vi "VI Tree.vi"   [LabVIEW 2016]
uses:
  Attributes.vi
  Error Code File Properties.ctl
  Error Owner and ID.ctl
  Error Owners and IDs.ctl
  Scope.ctl
types:
  T1 = typedef "Scope.ctl" = enum16{"project", "global"}
  T2 = typedef "Error Owners and IDs.ctl" = cluster{"owner path":string, "error IDs":string[]}
  T3 = typedef "Error Owner and ID.ctl" = cluster{"owner path":string, "ID":string}
  T4 = typedef "Error Code File Properties.ctl" = cluster{"path":path, "simplified path":string, "name":string, "display name":string, "family name":string, "comment":string, "parsable?":bool, "file modified?":bool}
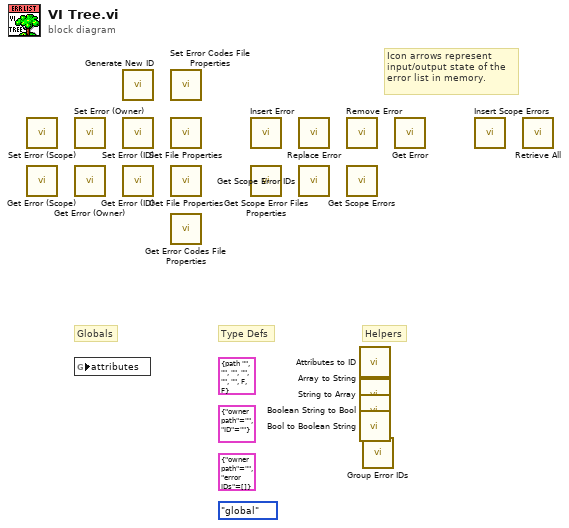
[diagram p0: block diagram]
diagram:
  (unwired) Scope."global" ("scope")
  (unwired) T2 {"owner path"="", "error IDs"=[]} ("error owners and IDs")
  (unwired) T3 {"owner path"="", "ID"=""} ("error owner and ID")
  (unwired) T4 {"path"=path "", "simplified path"="", "name"="", "display name"="", "family name"="", "comment"="", "parsable?"=FALSE, "file modified?"=FALSE} ("error code file properties")
  # "Icon arrows represent input/output state of the error list in memory."
  # "Globals"
  # "Type Defs"
  # "Helpers"
  n1 = call "Set Error (Scope).vi"() -> ()  [unwired: 10 in, 2 out]
  n2 = call "Get Error (Scope).vi"() -> ()  [unwired: 8 in, 4 out]
  n3 = call "Set Error (Owner).vi"() -> ()  [unwired: 10 in, 2 out]
  n4 = call "Get Error (Owner).vi"() -> ()  [unwired: 8 in, 4 out]
  n5 = global read "Attributes.vi" "attributes"() -> ()  [unwired: 1 in]
  n6 = call "Generate New ID.vi"() -> ()  [unwired: 9 in, 3 out]
  n7 = call "Set Error (ID).vi"() -> ()  [unwired: 10 in, 2 out]
  n8 = call "Get Error (ID).vi"() -> ()  [unwired: 7 in, 5 out]
  n9 = call "Set Error Codes File Properties.vi"() -> ()  [unwired: 10 in, 2 out]
  n10 = call "Set File Properties.vi"() -> ()  [unwired: 10 in, 2 out]
  n11 = call "Get File Properties.vi"() -> ()  [unwired: 9 in, 3 out]
  n12 = call "Get Error Codes File Properties.vi"() -> ()  [unwired: 8 in, 4 out]
  n13 = call "Insert Error.vi"() -> ()  [unwired: 10 in, 2 out]
  n14 = call "Get Scope Error Files Properties.vi"() -> ()  [unwired: 7 in, 5 out]
  n15 = call "Replace Error.vi"() -> ()  [unwired: 10 in, 2 out]
  n16 = call "Get Scope Error IDs.vi"() -> ()  [unwired: 9 in, 3 out]
  n17 = call "Remove Error.vi"() -> ()  [unwired: 10 in, 2 out]
  n18 = call "Get Scope Errors.vi"() -> ()  [unwired: 7 in, 5 out]
  n19 = call "Attributes to ID.vi"() -> ()  [unwired: 1 in, 1 out]
  n20 = call "Array to String.vi"() -> ()  [unwired: 2 in, 1 out]
  n21 = call "String to Array.vi"() -> ()  [unwired: 2 in, 1 out]
  n22 = call "Boolean String to Bool.vi"() -> ()  [unwired: 1 in, 1 out]
  n23 = call "Bool to Boolean String.vi"() -> ()  [unwired: 1 in, 1 out]
  n24 = call "Group Error IDs.vi"() -> ()  [unwired: 10 in, 2 out]
  n25 = call "Get Error.vi"() -> ()  [unwired: 7 in, 5 out]
  n26 = call "Insert Scope Errors.vi"() -> ()  [unwired: 10 in, 2 out]
  n27 = call "Retrieve All.vi"() -> ()  [unwired: 9 in, 3 out]
